vi "parseFormatedInput.vi"(10 "unit":string, 11 "inputString":string) -> (0 "matchValid":bool, 3 "parsedNumber":dbl)   [LabVIEW 2016, in "calibratedIOField.xctl"]
uses:
  calibratedIOField.xctl
panel:
  out "inputString 2":string
  out "concatenated string":string
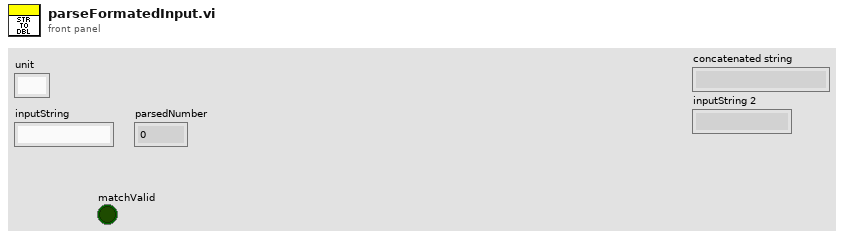
[diagram p1: front panel]
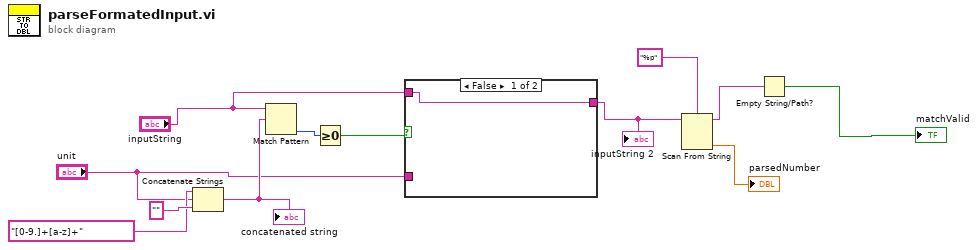
[diagram p0: block diagram]
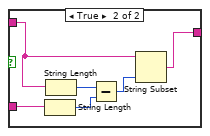
[diagram p2: hidden frame]
diagram:
  n1 = Concatenate Strings("[0-9.]+[a-z]+" ("regular expression"), "unit", "" ("string")) -> (w7:string)
  "concatenated string" <- w7
  n2 = Match Pattern(string="inputString", regular expression=w7) -> (offset past match=w11:i32)  [unwired: 1 in, 3 out]
  n3 = Greater Or Equal To 0?(x=w11) -> (x >= 0?=w10:bool)
  n4 = case shown="False" w10 {
    tunnel: "unit" -> [_ w18]
    tunnel: [w13 w15] -> w4
    tunnel: "inputString" -> [w13 w14]
    frame False {
    }
    frame True {
      n5 = String Length(string=w18) -> (length=w17:i32)
      n6 = String Length(string=w14) -> (length=w19:i32)
      n7 = Subtract(x=w19, y=w17) -> (x-y=w16:i32)
      n8 = String Subset(string=w14, length (rest)=w16) -> (substring=w15:string)  [unwired: 1 in]
    }
  }
  "inputString 2" <- w4
  n9 = Scan From String(format string="%p", input string=w4) -> (remaining string=w2:string, output 1=→"parsedNumber":dbl)  [unwired: 3 in, 2 out]
  n10 = Empty String/Path?(string/path=w2) -> (empty?=→"matchValid":bool)
